vi "Rohde & Schwarz VNA Sort Measurements.vi"(7 "Rohde & Schwarz VNA":T6, 8 "error in (no error)":errorcluster, 9 "Auto Select":bool, 10 "Parameters to Measure":T1[](array[typedef]) {"Channel" min=1 max=99 step=1; "Parameter"."Stimulus Port" min=1 step=1; "Parameter"."Response Port" min=1 step=1}, 11 "VISA Resource Name":refnum<visa-resource-name>) -> (0 "error out":errorcluster {"code" format="%.0x"}, 1 "Channels Used":i8[](array[numeric]), 2 "Sorted Measurements":cluster{"Measurements":T5[]}[](array[cluster]) {"Measurements"."Traces"."Parameter"."Stimulus Port" min=1 step=1; "Measurements"."Traces"."Parameter"."Response Port" min=1 step=1}, 3 "dup VISA Resource Name":refnum<visa-resource-name>, 4 "Sorted Parameters to Measure":T1[](array[typedef]) {"Channel" min=1 max=99 step=1; "Parameter"."Stimulus Port" min=1 step=1; "Parameter"."Response Port" min=1 step=1}, 5 "Removed Parameters":T1[](array[typedef]) {"Channel" min=1 max=99 step=1; "Parameter"."Stimulus Port" min=1 step=1; "Parameter"."Response Port" min=1 step=1}, 6 "Measurements Removed?":bool)   [LabVIEW 2011]
uses:
  tests/S Parameter/TypeDefs/SP Parameter to Measure.ctl
  tests/S Parameter/TypeDefs/SP Parameter.ctl
  tests/S Parameter/TypeDefs/SP Calibration State.ctl
  tests/S Parameter/TypeDefs/SP Measurement Format.ctl
  TypeDefs/Rohde & Schwarz VNA Instrument Info.ctl
  Agilent/TypeDefs/Agilent VNA Measurements.ctl
  Summitek/Win32/Miscellaneous/Add to Array if Not Present (I32).vi
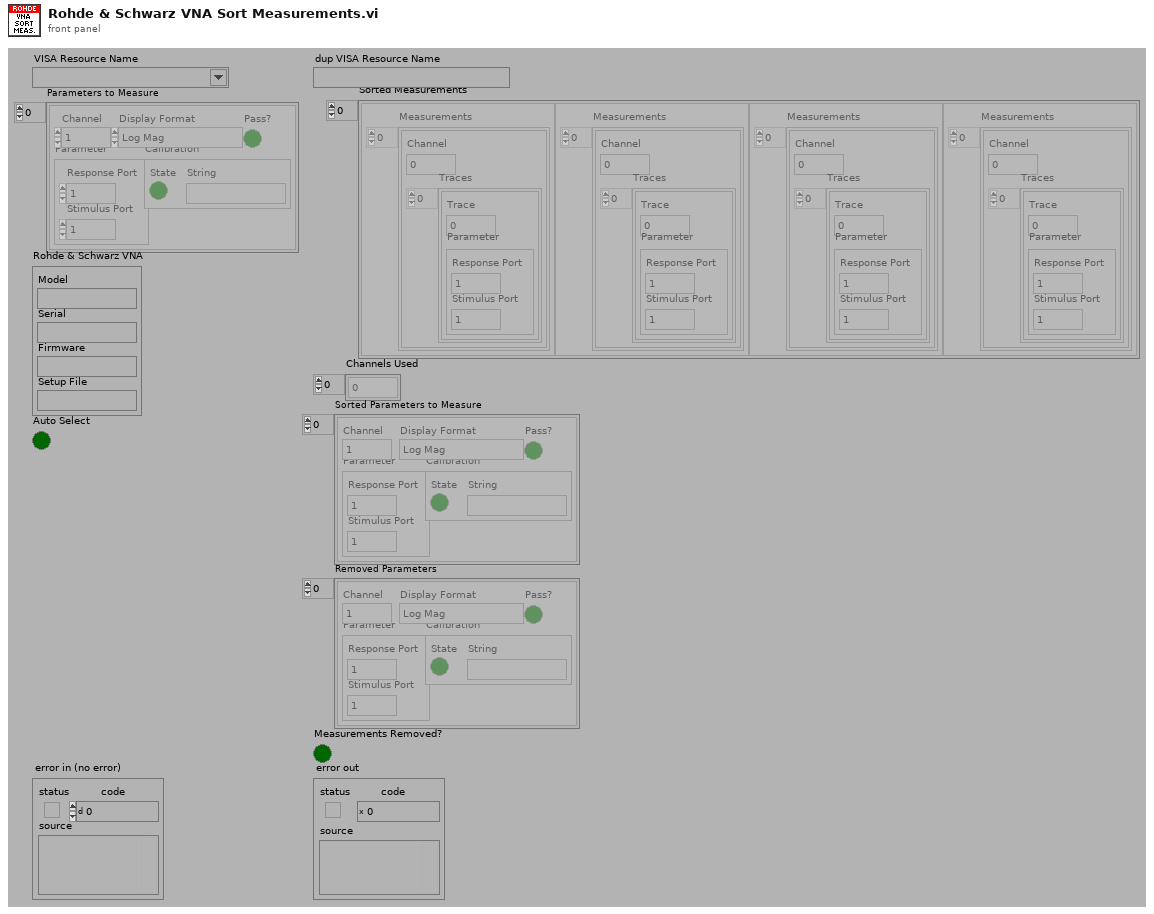
[diagram p1: front panel]
types:
  T1 = typedef "SP Parameter to Measure.ctl" = cluster{"Channel":i8, "Parameter":T2, "Calibration":T3, "Display Format":T4, "Pass?":bool}
  T2 = typedef "SP Parameter.ctl" = cluster{"Stimulus Port":i8, "Response Port":i8}
  T3 = typedef "SP Calibration State.ctl" = cluster{"State":bool, "String":string}
  T4 = typedef "SP Measurement Format.ctl" = enum32{"Log Mag", "Phase", "Delay", "Smith (R+jX)", "Polar (Re/Im)", "Linear Mag", "SWR", "Real", "Imaginary", "Smith (Lin/Phase)", "Smith (Log/Phase)", "Smith (Real/Imag)", "Smith (G+jB)", "Polar (Lin/Phase)", "Polar (Log/Phase)", "Expanded Phase", "Positive Phase", "Inverted Smith", "Unwrapped Phase", "Power Out", "Power In", "Linear Mag/Phase", "Log Mag/Phase", "Real/Imaginary"}
  T5 = typedef "Agilent VNA Measurements.ctl" = cluster{"Channel":i8, "Traces":cluster{"Trace":i8, "Parameter":T2}[]}
  T6 = typedef "Rohde & Schwarz VNA Instrument Info.ctl" = cluster{"Model":string, "Serial":string, "Firmware":string, "Setup File":string}
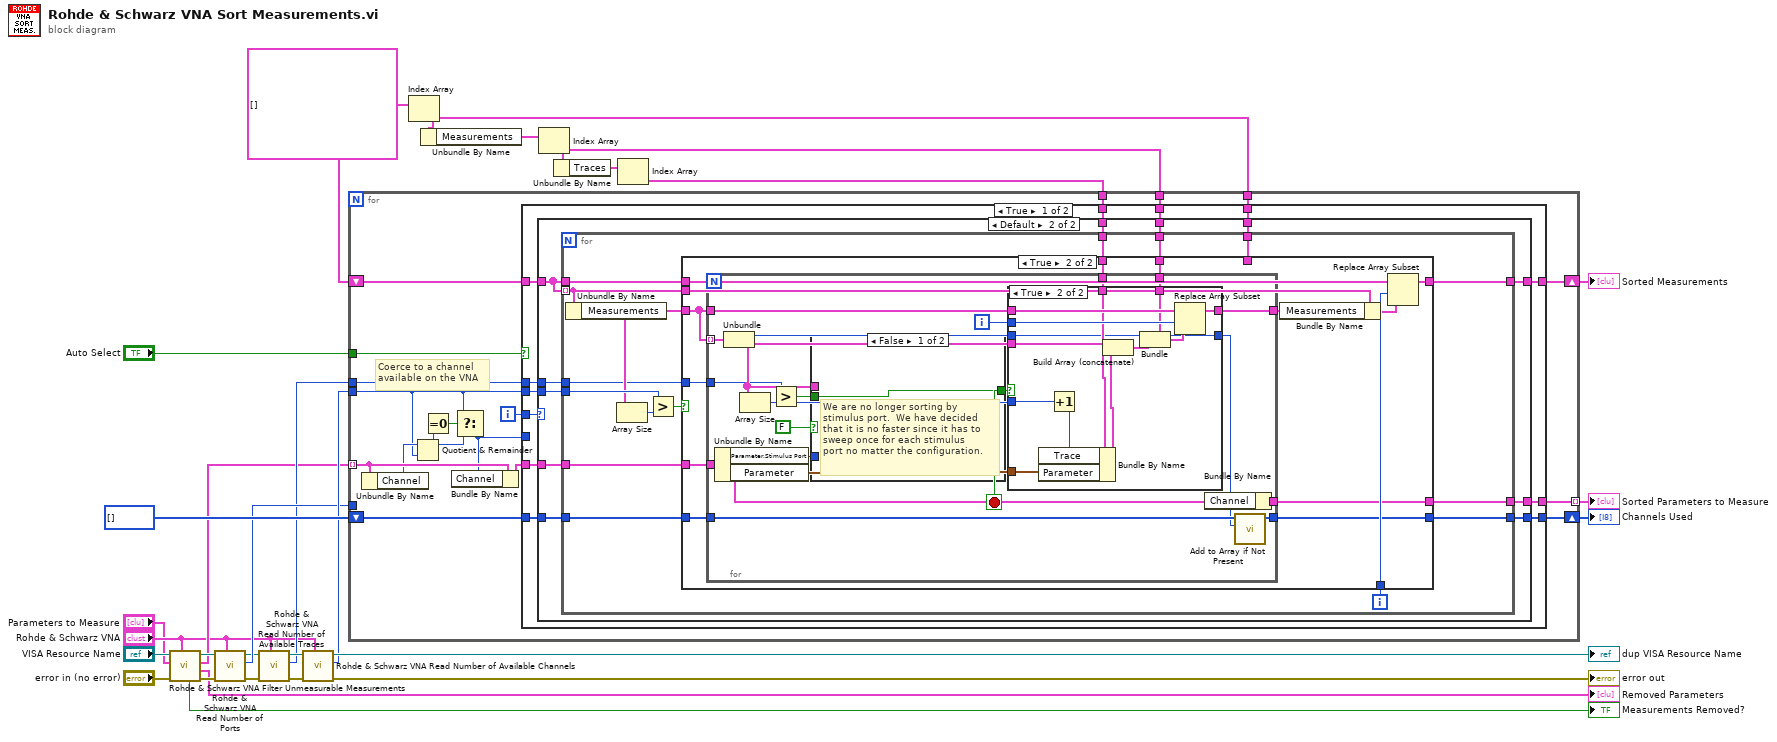
[diagram p0: block diagram]
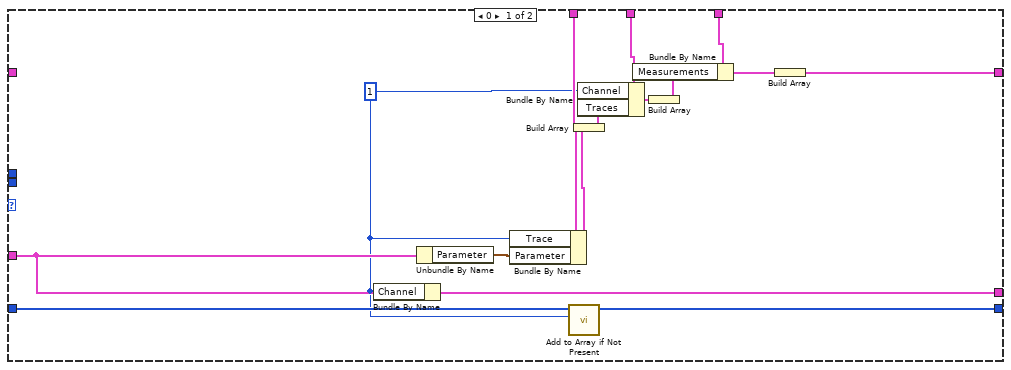
[diagram p2: hidden frame]
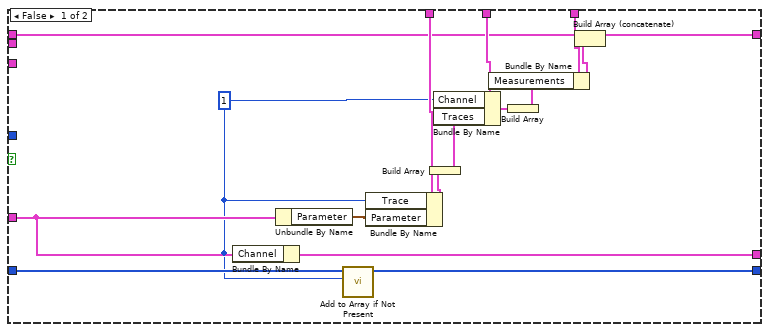
[diagram p3: hidden frame]
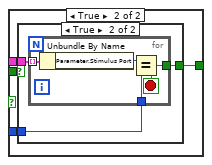
[diagram p4: hidden frame]
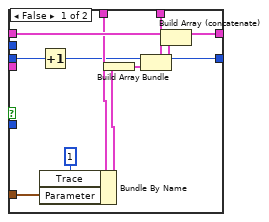
[diagram p6: hidden frame]
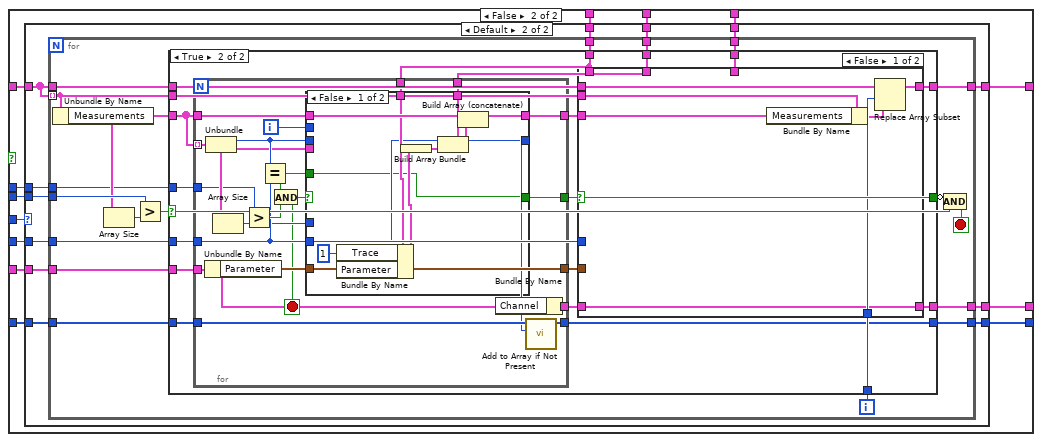
[diagram p7: hidden frame]
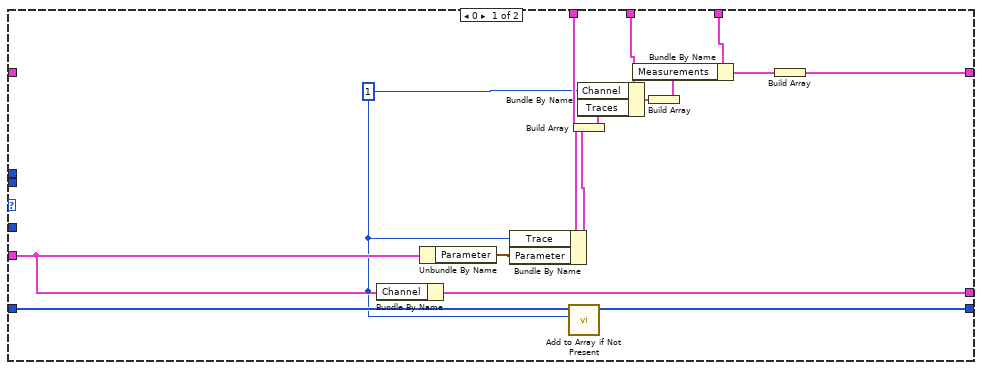
[diagram p8: hidden frame]
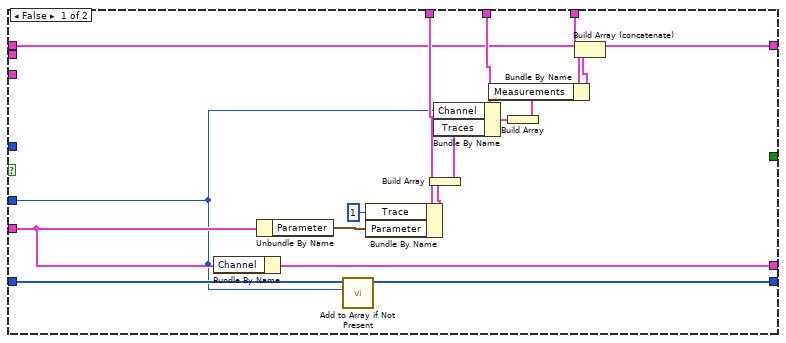
[diagram p9: hidden frame]
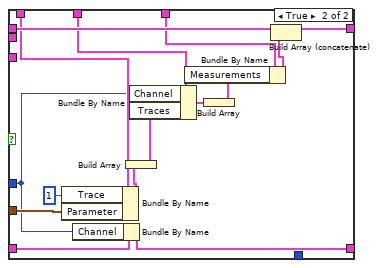
[diagram p10: hidden frame]
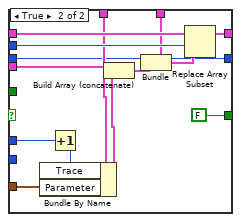
[diagram p11: hidden frame]
diagram:
  w24 = cluster{"Measurements":T5[]}[] [] ("Sorted Measurements")
  n1 = call "Rohde & Schwarz VNA Filter Unmeasurable Measurements.vi"("Rohde & Schwarz VNA"="Rohde & Schwarz VNA", "error in (no error)"="error in (no error)", "Parameters to Measure"="Parameters to Measure", "VISA Resource Name"="VISA Resource Name") -> ("error out"=w10:errorcluster, "Removed Parameters"=→"Removed Parameters":T1[], "Filtered Parameters to Measure"=w6:T1[], "dup VISA Resource Name"=w9:refnum<visa-resource-name>, "Measurements Removed?"=→"Measurements Removed?":bool)  [unwired: 3 out]
  n2 = call "Rohde & Schwarz VNA Read Number of Ports.vi"("Rohde & Schwarz VNA"="Rohde & Schwarz VNA", "error in (no error)"=w10, "VISA Resource Name"=w9) -> ("error out"=w14:errorcluster, "Number of Ports"=w16:i8, "dup VISA Resource Name"=w15:refnum<visa-resource-name>)  [unwired: 6 out]
  n3 = call "Rohde & Schwarz VNA Read Number of Available Traces.vi"("Rohde & Schwarz VNA"="Rohde & Schwarz VNA", "error in (no error)"=w14, "VISA Resource Name"=w15) -> ("error out"=w13:errorcluster, "Number of Traces"=w11:i8, "dup VISA Resource Name"=w12:refnum<visa-resource-name>)  [unwired: 6 out]
  n4 = call "Rohde & Schwarz VNA Read Number of Available Channels.vi"("Rohde & Schwarz VNA"="Rohde & Schwarz VNA", "error in (no error)"=w13, "VISA Resource Name"=w12) -> ("error out"=→"error out":errorcluster, "Number of Channels"=w17:i8, "dup VISA Resource Name"=→"dup VISA Resource Name":refnum<visa-resource-name>)  [unwired: 6 out]
  n5 = Index Array(array=w24) -> (element=w20:cluster{"Measurements":T5[]})  [unwired: 1 in]
  n6 = Unbundle By Name(w20) -> ("Measurements"=w26:T5[])
  n7 = Index Array(array=w26) -> (element=w21:T5)  [unwired: 1 in]
  n8 = Unbundle By Name(w21) -> ("Traces"=w23:cluster{"Trace":i8, "Parameter":T2}[])
  n9 = Index Array(array=w23) -> (element=w22:cluster{"Trace":i8, "Parameter":T2})  [unwired: 1 in]
  n10 = for {
    tunnel: w6 -> [w45] mode=indexing
    shift-right: [w35] -> w25
    shift-left: w24 -> [w46]
    tunnel: w17 -> [w40]
    tunnel: "Auto Select" -> [w38]
    tunnel: w22 -> [w37]
    tunnel: w21 -> [w36]
    tunnel: w20 -> [w34]
    shift-right: [w32] -> w18
    shift-left: i8[] [] -> [w33]
    tunnel: w16 -> [_]
    tunnel: w11 -> [w31]
    tunnel: [w30] -> w1 mode=indexing
    i -> [w47]
    # "Coerce to a channel\navailable on the VNA"
    n11 = Unbundle By Name(w45) -> ("Channel"=w43:i8)
    n12 = Quotient & Remainder(x=w43, y=w40) -> (x-y*floor(x/y)=w39:i8)  [unwired: 1 out]
    n13 = Equal To 0?(x=w39) -> (x = 0?=w42:bool)
    n14 = Select(t=w40, s=w42, f=w39) -> (s? t:f=w41:i8)
    n15 = Bundle By Name(cluster=w45, "Channel"=w41) -> (w44:T1)
    n16 = case shown="True" w38 {
      tunnel: w47 -> [w53 w195]
      tunnel: w46 -> [w59 w201]
      tunnel: w44 -> [w58 w200]
      tunnel: w41 -> [_ w191]
      tunnel: w40 -> [w57 w199]
      tunnel: w37 -> [w56 w198]
      tunnel: w36 -> [w55 w197]
      tunnel: [w54 w196] -> w35
      tunnel: w34 -> [w52 w194]
      tunnel: w33 -> [w51 w193]
      tunnel: [w50 w192] -> w32
      tunnel: w31 -> [w49 w190]
      tunnel: [w48 w189] -> w30
      frame True {
        n17 = case shown="Default" w53 {
          tunnel: w59 -> [_ w80]
          tunnel: w58 -> [w62 w85]
          tunnel: w57 -> [_ w84]
          tunnel: w56 -> [w74 w83]
          tunnel: w55 -> [w72 w82]
          tunnel: [w65 w81] -> w54
          tunnel: w52 -> [w68 w79]
          tunnel: w51 -> [w64 w78]
          tunnel: [w63 w77] -> w50
          tunnel: w49 -> [_ w76]
          tunnel: [w61 w75] -> w48
          frame 0 {
            w60 = i8 1 ("Channel")
            n18 = Bundle By Name(cluster=w62, "Channel"=w60) -> (w61:T1)
            n19 = Unbundle By Name(w62) -> ("Parameter"=w73:T2)
            n20 = Bundle By Name(cluster=w74, "Trace"=w60, "Parameter"=w73) -> (w70:cluster{"Trace":i8, "Parameter":T2})
            n21 = call-poly "Add to Array if Not Present.vi"("I32"=w60, "I32 Array"=w64) -> ("New I32 Array"=w63:i32[])  [unwired: 3 out]
            n22 = Build Array(w70) -> (w69:cluster{"Trace":i8, "Parameter":T2}[])
            n23 = Bundle By Name(cluster=w72, "Channel"=w60, "Traces"=w69) -> (w71:T5)
            n24 = Build Array(w71) -> (w67:T5[])
            n25 = Bundle By Name(cluster=w68, "Measurements"=w67) -> (w66:cluster{"Measurements":T5[]})
            n26 = Build Array(w66) -> (w65:cluster{"Measurements":T5[]}[])
          }
          frame Default {
            n27 = for {
              tunnel: w80 -> [w94]
              tunnel: w85 -> [w101]
              tunnel: w84 -> [w97]
              tunnel: w83 -> [w100]
              tunnel: w82 -> [w99]
              tunnel: [w98] -> w81
              tunnel: w80 -> [w90] mode=indexing
              tunnel: w79 -> [w91]
              tunnel: w78 -> [w89]
              tunnel: [w88] -> w77
              tunnel: w76 -> [w87]
              tunnel: [w86] -> w75
              i -> [w93]
              n28 = Unbundle By Name(w90) -> ("Measurements"=w92:T5[])
              n29 = Array Size(array=w92) -> (size(s)=w96:i32)
              n30 = Greater?(x=w97, y=w96) -> (0:w95:bool)
              n31 = case shown="True" w95 {
                tunnel: w101 -> [w103 w131]
                tunnel: w100 -> [w115 w130]
                tunnel: w99 -> [w114 w129]
                tunnel: [w117 w126] -> w98
                tunnel: w92 -> [_ w128]
                tunnel: w94 -> [w111 w127]
                tunnel: w93 -> [_ w125]
                tunnel: w91 -> [w109 _]
                tunnel: w90 -> [_ w124]
                tunnel: w89 -> [w106 w121]
                tunnel: [w105 w120] -> w88
                tunnel: w87 -> [_ w119]
                tunnel: [w104 w118] -> w86
                frame False {
                  w102 = i8 1 ("Channel")
                  n32 = Bundle By Name(cluster=w103, "Channel"=w102) -> (w104:T1)
                  n33 = Unbundle By Name(w103) -> ("Parameter"=w116:T2)
                  n34 = call-poly "Add to Array if Not Present.vi"("I32"=w102, "I32 Array"=w106) -> ("New I32 Array"=w105:i32[])  [unwired: 3 out]
                  n35 = Bundle By Name(cluster=w115, "Trace"=w102, "Parameter"=w116) -> (w113:cluster{"Trace":i8, "Parameter":T2})
                  n36 = Build Array(w113) -> (w112:cluster{"Trace":i8, "Parameter":T2}[])
                  n37 = Bundle By Name(cluster=w114, "Channel"=w102, "Traces"=w112) -> (w110:T5)
                  n38 = Build Array(w110) -> (w108:T5[])
                  n39 = Bundle By Name(cluster=w109, "Measurements"=w108) -> (w107:cluster{"Measurements":T5[]})
                  n40 = Build Array (concatenate)(w111, w107) -> (w117:cluster{"Measurements":T5[]}[])
                }
                frame True {
                  n41 = for {
                    tunnel: w128 -> [w147] mode=indexing
                    tunnel: w131 -> [w133]
                    tunnel: w128 -> [w151]
                    tunnel: [w148] -> w123
                    tunnel: w130 -> [w143]
                    tunnel: w129 -> [w141]
                    tunnel: w121 -> [w138]
                    tunnel: [w137] -> w120
                    tunnel: w119 -> [w136]
                    tunnel: [w134] -> w118
                    i -> [w150]
                    stop <- w146 stop-if-true
                    n42 = Unbundle By Name(w133) -> ("Parameter.Stimulus Port"=w139:i8, "Parameter"=w140:T2)
                    n43 = Unbundle(w147) -> ("Channel"=w144:i8, "Traces"=w145:cluster{"Trace":i8, "Parameter":T2}[])
                    n44 = Array Size(array=w145) -> (size(s)=w142:i32)
                    n45 = Greater?(x=w136, y=w142) -> (0:w149:bool)
                    n46 = case shown="False" FALSE {
                      tunnel: w149 -> [w152 w156]
                      tunnel: [w152 w155] -> w146
                      tunnel: w145 -> [_ w154]
                      tunnel: w139 -> [_ w153]
                      frame False {
                        # "We are no longer sorting by\nstimulus port.  We have decided\nthat it is no faster since it has to\nsweep once for each stimulus\nport no matter the configuration."
                      }
                      frame True {
                        n47 = case shown="True" w156 {
                          selector: w156 -> [w157 _]
                          tunnel: w154 -> [_ w160]
                          tunnel: [w157 w159] -> w155
                          tunnel: w153 -> [_ w158]
                          frame False {
                          }
                          frame True {
                            n48 = for {
                              tunnel: w160 -> [w164] mode=indexing
                              tunnel: [w162] -> w159
                              tunnel: w158 -> [w161]
                              stop <- w162 stop-if-true
                              n49 = Unbundle By Name(w164) -> ("Parameter.Stimulus Port"=w163:i8)
                              n50 = Equal?(x=w163, y=w161) -> (x = y?=w162:bool)
                            }
                          }
                        }
                      }
                    }
                    n51 = case shown="True" w146 {
                      tunnel: w145 -> [_ w184]
                      tunnel: w151 -> [w175 w188]
                      tunnel: w150 -> [_ w187]
                      tunnel: [w174 w186] -> w148
                      tunnel: w144 -> [w167 w176]
                      tunnel: w140 -> [w170 w182]
                      tunnel: w143 -> [w169 w183]
                      tunnel: w142 -> [_ w181]
                      tunnel: w141 -> [w171 w178]
                      tunnel: [w165 w176] -> w135
                      frame False {
                        n52 = Increment(x=w167) -> (x+1=w165:i8)
                        n53 = Bundle By Name(cluster=w169, "Trace"=i8 1, "Parameter"=w170) -> (w168:cluster{"Trace":i8, "Parameter":T2})
                        n54 = Build Array(w168) -> (w172:cluster{"Trace":i8, "Parameter":T2}[])
                        n55 = Bundle(cluster=w171, "Channel"=w165, "Traces"=w172) -> (w173:T5)
                        n56 = Build Array (concatenate)(w175, w173) -> (w174:T5[])
                      }
                      frame True {
                        n57 = Increment(x=w181) -> (x+1=w180:i32)
                        n58 = Bundle By Name(cluster=w183, "Trace"=w180, "Parameter"=w182) -> (w179:cluster{"Trace":i8, "Parameter":T2})
                        n59 = Build Array (concatenate)(w184, w179) -> (w177:cluster{"Trace":i8, "Parameter":T2}[])
                        n60 = Bundle(cluster=w178, "Channel"=w176, "Traces"=w177) -> (w185:T5)
                        n61 = Replace Array Subset(array=w188, new element=w185, index=w187) -> (w186:T5[])
                      }
                    }
                    n62 = Bundle By Name(cluster=w133, "Channel"=w135) -> (w134:T1)
                    n63 = call-poly "Add to Array if Not Present.vi"("I32"=w135, "I32 Array"=w138) -> ("New I32 Array"=w137:i32[])  [unwired: 3 out]
                  }
                  n64 = Bundle By Name(cluster=w124, "Measurements"=w123) -> (w122:cluster{"Measurements":T5[]})
                  n65 = Replace Array Subset(array=w127, new element=w122, index=w125) -> (w126:cluster{"Measurements":T5[]}[])
                }
              }
            }
          }
        }
      }
      frame False {
        n66 = case shown="Default" w195 {
          tunnel: w201 -> [_ w223]
          tunnel: w200 -> [w204 w228]
          tunnel: w199 -> [_ w227]
          tunnel: w198 -> [w216 w226]
          tunnel: w197 -> [w214 w225]
          tunnel: [w207 w224] -> w196
          tunnel: w194 -> [w210 w222]
          tunnel: w193 -> [w206 w221]
          tunnel: [w205 w220] -> w192
          tunnel: w191 -> [_ w219]
          tunnel: w190 -> [_ w218]
          tunnel: [w203 w217] -> w189
          frame 0 {
            w202 = i8 1 ("Channel")
            n67 = Bundle By Name(cluster=w204, "Channel"=w202) -> (w203:T1)
            n68 = Unbundle By Name(w204) -> ("Parameter"=w215:T2)
            n69 = Bundle By Name(cluster=w216, "Trace"=w202, "Parameter"=w215) -> (w212:cluster{"Trace":i8, "Parameter":T2})
            n70 = call-poly "Add to Array if Not Present.vi"("I32"=w202, "I32 Array"=w206) -> ("New I32 Array"=w205:i32[])  [unwired: 3 out]
            n71 = Build Array(w212) -> (w211:cluster{"Trace":i8, "Parameter":T2}[])
            n72 = Bundle By Name(cluster=w214, "Channel"=w202, "Traces"=w211) -> (w213:T5)
            n73 = Build Array(w213) -> (w209:T5[])
            n74 = Bundle By Name(cluster=w210, "Measurements"=w209) -> (w208:cluster{"Measurements":T5[]})
            n75 = Build Array(w208) -> (w207:cluster{"Measurements":T5[]}[])
          }
          frame Default {
            n76 = for {
              tunnel: w223 -> [w241]
              tunnel: w228 -> [w247]
              tunnel: w227 -> [w243]
              tunnel: w226 -> [w246]
              tunnel: w225 -> [w245]
              tunnel: [w244] -> w224
              tunnel: w223 -> [w237] mode=indexing
              tunnel: w222 -> [w238]
              tunnel: w221 -> [w236]
              tunnel: [w235] -> w220
              tunnel: w219 -> [w234]
              tunnel: w218 -> [w230]
              tunnel: [w229] -> w217
              i -> [w240]
              stop <- w231 stop-if-true
              n77 = Unbundle By Name(w237) -> ("Measurements"=w239:T5[])
              n78 = Array Size(array=w239) -> (size(s)=w242:i32)
              n79 = Greater?(x=w243, y=w242) -> (0:w232:bool)
              n80 = case shown="True" w232 {
                tunnel: w247 -> [w250 w282]
                tunnel: w246 -> [w262 w273]
                tunnel: w245 -> [w261 w272]
                tunnel: [w264 w279] -> w244
                tunnel: w239 -> [_ w281]
                tunnel: w241 -> [w258 w280]
                tunnel: w240 -> [_ w278]
                tunnel: w238 -> [w256 w269]
                tunnel: w237 -> [_ w277]
                tunnel: w236 -> [w253 w275]
                tunnel: [w252 w274] -> w235
                tunnel: w234 -> [w248 w270]
                tunnel: [_ w268] -> w233
                tunnel: w230 -> [_ w267]
                tunnel: [w249 w265] -> w229
                frame False {
                  n81 = Bundle By Name(cluster=w250, "Channel"=w248) -> (w249:T1)
                  n82 = Unbundle By Name(w250) -> ("Parameter"=w263:T2)
                  n83 = call-poly "Add to Array if Not Present.vi"("I32"=w248, "I32 Array"=w253) -> ("New I32 Array"=w252:i32[])  [unwired: 3 out]
                  n84 = Bundle By Name(cluster=w262, "Trace"=i8 1 ("Channel"), "Parameter"=w263) -> (w260:cluster{"Trace":i8, "Parameter":T2})
                  n85 = Build Array(w260) -> (w259:cluster{"Trace":i8, "Parameter":T2}[])
                  n86 = Bundle By Name(cluster=w261, "Channel"=w248, "Traces"=w259) -> (w257:T5)
                  n87 = Build Array(w257) -> (w255:T5[])
                  n88 = Bundle By Name(cluster=w256, "Measurements"=w255) -> (w254:cluster{"Measurements":T5[]})
                  n89 = Build Array (concatenate)(w258, w254) -> (w264:cluster{"Measurements":T5[]}[])
                }
                frame True {
                  n90 = for {
                    tunnel: w281 -> [w322] mode=indexing
                    tunnel: w282 -> [w307]
                    tunnel: w281 -> [w325]
                    tunnel: [w323] -> w276
                    tunnel: w273 -> [w321]
                    tunnel: w272 -> [w320]
                    tunnel: w275 -> [w319]
                    tunnel: [w318] -> w274
                    tunnel: w270 -> [w313]
                    tunnel: [w316] -> w271
                    tunnel: [w310] -> w268
                    tunnel: w267 -> [w308]
                    tunnel: [w306] -> w266
                    i -> [w324]
                    stop <- w311 stop-if-true
                    n91 = Unbundle By Name(w307) -> ("Parameter"=w316:T2)
                    n92 = Unbundle(w322) -> ("Channel"=w317:i8, "Traces"=w315:cluster{"Trace":i8, "Parameter":T2}[])
                    n93 = Array Size(array=w315) -> (size(s)=w312:i32)
                    n94 = Greater?(x=w308, y=w312) -> (0:w314:bool)
                    n95 = Equal?(x=w317, y=w313) -> (x = y?=w309:bool)
                    n96 = And(x=w309, y=w314) -> (x .and. y?=w311:bool)
                    n97 = case shown="False" w311 {
                      tunnel: w315 -> [_ w346]
                      tunnel: w325 -> [w336 w350]
                      tunnel: w324 -> [_ w349]
                      tunnel: [w335 w348] -> w323
                      tunnel: w317 -> [_ w340]
                      tunnel: w316 -> [w329 w344]
                      tunnel: w321 -> [w331 w345]
                      tunnel: w320 -> [w332 w342]
                      tunnel: [w327 w340] -> w305
                      tunnel: w313 -> [w327 _]
                      tunnel: w312 -> [_ w339]
                      tunnel: [w326 FALSE] -> w310
                      tunnel: w309 -> [w326 _]
                      frame False {
                        n98 = Bundle By Name(cluster=w331, "Trace"=i8 1, "Parameter"=w329) -> (w330:cluster{"Trace":i8, "Parameter":T2})
                        n99 = Build Array(w330) -> (w333:cluster{"Trace":i8, "Parameter":T2}[])
                        n100 = Bundle(cluster=w332, "Channel"=w327, "Traces"=w333) -> (w334:T5)
                        n101 = Build Array (concatenate)(w336, w334) -> (w335:T5[])
                      }
                      frame True {
                        n102 = Increment(x=w339) -> (x+1=w338:i32)
                        n103 = Bundle By Name(cluster=w345, "Trace"=w338, "Parameter"=w344) -> (w343:cluster{"Trace":i8, "Parameter":T2})
                        n104 = Build Array (concatenate)(w346, w343) -> (w341:cluster{"Trace":i8, "Parameter":T2}[])
                        n105 = Bundle(cluster=w342, "Channel"=w340, "Traces"=w341) -> (w347:T5)
                        n106 = Replace Array Subset(array=w350, new element=w347, index=w349) -> (w348:T5[])
                      }
                    }
                    n107 = Bundle By Name(cluster=w307, "Channel"=w305) -> (w306:T1)
                    n108 = call-poly "Add to Array if Not Present.vi"("I32"=w305, "I32 Array"=w319) -> ("New I32 Array"=w318:i32[])  [unwired: 3 out]
                  }
                  n109 = case shown="False" w268 {
                    tunnel: w280 -> [w289 w298]
                    tunnel: [w288 w297] -> w279
                    tunnel: w278 -> [w287 _]
                    tunnel: w277 -> [w286 _]
                    tunnel: w276 -> [w285 _]
                    tunnel: w273 -> [_ w296]
                    tunnel: w272 -> [_ w294]
                    tunnel: w271 -> [_ w295]
                    tunnel: w270 -> [_ w290]
                    tunnel: w269 -> [_ w293]
                    tunnel: w266 -> [w283 w292]
                    tunnel: [w283 w291] -> w265
                    frame False {
                      n110 = Bundle By Name(cluster=w286, "Measurements"=w285) -> (w284:cluster{"Measurements":T5[]})
                      n111 = Replace Array Subset(array=w289, new element=w284, index=w287) -> (w288:cluster{"Measurements":T5[]}[])
                    }
                    frame True {
                      n112 = Bundle By Name(cluster=w296, "Trace"=i8 1 ("Channel"), "Parameter"=w295) -> (w304:cluster{"Trace":i8, "Parameter":T2})
                      n113 = Bundle By Name(cluster=w292, "Channel"=w290) -> (w291:T1)
                      n114 = Build Array(w304) -> (w303:cluster{"Trace":i8, "Parameter":T2}[])
                      n115 = Bundle By Name(cluster=w294, "Channel"=w290, "Traces"=w303) -> (w302:T5)
                      n116 = Build Array(w302) -> (w301:T5[])
                      n117 = Bundle By Name(cluster=w293, "Measurements"=w301) -> (w300:cluster{"Measurements":T5[]})
                      n118 = Build Array (concatenate)(w298, w300) -> (w297:cluster{"Measurements":T5[]}[])
                    }
                  }
                }
              }
              n119 = Compound Arithmetic op=AND(invert w233, w232) -> (w231:bool)
            }
          }
        }
      }
    }
  }
  "Sorted Measurements" <- w25
  "Channels Used" <- w18
  "Sorted Parameters to Measure" <- w1
